vi "Ramp Speeds.vi"() -> ()   [LabVIEW 2009, in "Magnet.lvclass"]
uses:
  Magnet.lvclass
panel:
  out "Array":dbl[][](array[numeric])=[[0.342, 5.0, 1.0, 14.604], [0.137, 2.0, 1.0, 14.604], [0.068, 1.0, 1.0, 14.604], [0.068, 1.0, 0.5, 7.302]]
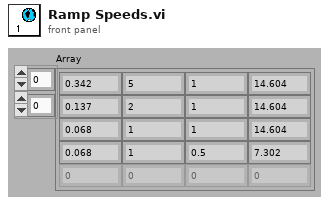
[diagram p1: front panel]
diagram:
